vi "status of power_supply2.vi"() -> ()   [LabVIEW 2020]
panel:
  out "status of power_supply2":bool
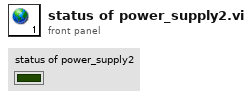
[diagram p1: front panel]
diagram:
